vi "Cocker.vi"(10 "Position":enum16{"Forward", "Reverse"}(ring)) -> (2 "In Position":bool)   [LabVIEW 2013]
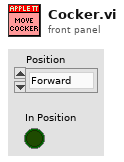
[diagram p1: front panel]
types:
  T1 = typedef "WPI_DigitalInputDevRef.ctl" = cluster{"DevStatus":errorcluster, "DIO Channel":T2, "Digital Module":T3}
  T2 = typedef "FPGA_DIOChannel.ctl" = enum8{"DIO 1", "DIO 2", "DIO 3", "DIO 4", "DIO 5", "DIO 6", "DIO 7", "DIO 8", "DIO 9", "DIO 10", "DIO 11", "DIO 12", "DIO 13", "DIO 14", "Invalid"}
  T3 = typedef "FPGA_TypedefDigitalModule.ctl" = enum16{"Digital Module 1", "Digital Module 2"}
  T4 = typedef "WPI_EncoderDevRef.ctl" = cluster{"DevStatus":errorcluster, "EncoderIndex":T5, "CounterIndex":T6, "DistancePerCount":dbl, "Decoding Type":T7}
  T5 = typedef "FPGA_EncoderIdx.ctl" = enum8{"Enc 0", "Enc 1", "Enc 2", "Enc 3", "Invalid"}
  T6 = typedef "FPGA_CounterCtrSystemIndex.ctl" = enum8{"Ctr 0", "Ctr 1", "Ctr 2", "Ctr 3", "Ctr 4", "Ctr 5", "Ctr 6", "Ctr 7", "Invalid"}
  T7 = typedef "WPI_EncoderType.ctl" = enum16{"1x", "2x", "4x"}
  T8 = typedef "WPI_MotorControlDeviceRef.ctl" = cluster{"DeviceStatus":errorcluster, "Type":enum16{"PWM", "CAN"}, "PWM":cluster{"Digital Module":T3, "PWM Channel":T9, "DeadBand":T10}, "CAN":cluster{"Device Number":u8, "Control Mode":T11, "Semaphore":T12, "Max Vout":dbl}, "Invert":bool, "TransformRef":T13, "InvTransformRef":T13}
  T9 = typedef "FPGA_DIOPWMChannel.ctl" = enum8{"PWM 1", "PWM 2", "PWM 3", "PWM 4", "PWM 5", "PWM 6", "PWM 7", "PWM 8", "PWM 9", "PWM 10", "Invalid"}
  T10 = typedef "WPI_PWMDeadband.ctl" = cluster{"Name":string, "maxPositivePwm":i32, "minPositivePwm":i32, "centerPwm":i32, "maxNegativePwm":i32, "minNegativePwm":i32, "angularRange":u16}
  T11 = typedef "WPI_CANJaguar_ControlMode.ctl" = enum8{"Percent VBus", "Current", "Speed", "Position", "Voltage"}
  T12 = typedef "Semaphore RefNum" = refnum<k1>
  T13 = typedef "WPI_PWMTransform_ConPane.ctl" = refnum<vi>
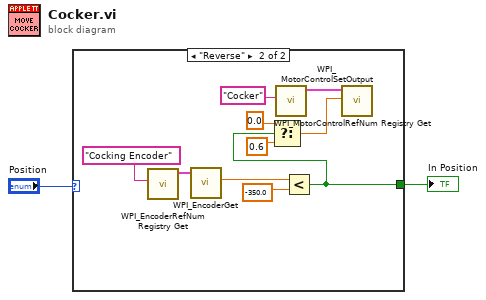
[diagram p0: block diagram]
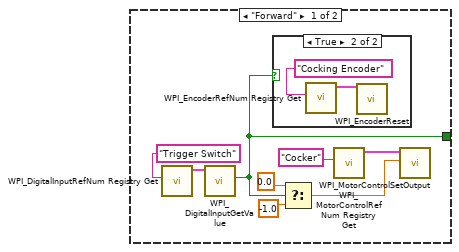
[diagram p2: hidden frame]
diagram:
  n1 = case shown="\"Reverse\"" "Position" {
    tunnel: [w5 w13] -> w1
    frame "Forward" {
      n2 = call <vilib>:"WPI_DigitalInputRefNum Registry Get.vi"("refnum name"="Trigger Switch") -> ("DigitalInputDevRef"=w10:T1)  [unwired: 9 in, 1 out]
      n3 = call <vilib>:"WPI_DigitalInputGetValue.vi"("DigitalInputDevRef"=w10) -> ("Value"=w5:bool)  [unwired: 8 in, 2 out]
      n4 = case shown="True" w5 {
        frame False {
        }
        frame True {
          n5 = call <vilib>:"WPI_EncoderRefNum Registry Get.vi"("refnum name"="Cocking Encoder") -> ("EncoderDevRef"=w11:T4)  [unwired: 9 in, 1 out]
          n6 = call <vilib>:"WPI_EncoderReset.vi"("EncoderDevRef"=w11) -> ()  [unwired: 9 in, 2 out]
        }
      }
      n7 = Select(t=0.0, s=w5, f=-1.0) -> (s? t:f=w3:dbl)
      n8 = call <vilib>:"WPI_MotorControlRefNum Registry Get.vi"("refnum name"="Cocker") -> ("MotorControlDevRef"=w7:T8)  [unwired: 9 in, 1 out]
      n9 = call <vilib>:"WPI_MotorControlSetOutput.vi"("Output"=w3, "MotorControlDevRef"=w7) -> ()  [unwired: 7 in, 3 out]
    }
    frame "Reverse" {
      n10 = call <vilib>:"WPI_EncoderRefNum Registry Get.vi"("refnum name"="Cocking Encoder") -> ("EncoderDevRef"=w21:T4)  [unwired: 9 in, 1 out]
      n11 = call <vilib>:"WPI_EncoderGet.vi"("EncoderDevRef"=w21) -> ("Distance"=w20:dbl)  [unwired: 5 in, 5 out]
      n12 = call <vilib>:"WPI_MotorControlRefNum Registry Get.vi"("refnum name"="Cocker") -> ("MotorControlDevRef"=w17:T8)  [unwired: 9 in, 1 out]
      n13 = Less?(x=w20, y=-350.0) -> (x < y?=w13:bool)
      n14 = Select(t=0.0, s=w13, f=0.6) -> (s? t:f=w14:dbl)
      n15 = call <vilib>:"WPI_MotorControlSetOutput.vi"("Output"=w14, "MotorControlDevRef"=w17) -> ()  [unwired: 7 in, 3 out]
    }
  }
  "In Position" <- w1
